vi "Colors.vi"() -> (0 "Highlight Color":u32(colorbox)=16776960, 1 "Text Color":u32(colorbox)=12303291, 2 "GridView Normal Color":u32(colorbox)=3618615, 3 "GridView Mouseover Color":u32(colorbox)=6645093)   [LabVIEW 2012, in "Win8uiFramework.lvlib"]
uses:
  Win8uiFramework/Win8uiFramework.lvlib
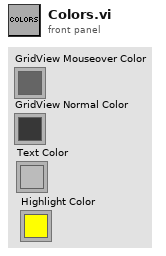
[diagram p1: front panel]
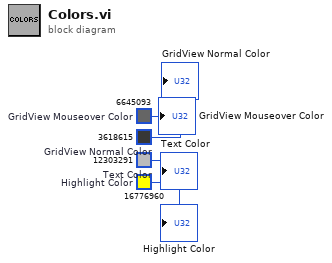
[diagram p0: block diagram]
diagram:
  w3 = u32 3618615  # GridView Normal Color
  w1 = u32 16776960  # Highlight Color
  w2 = u32 12303291  # Text Color
  w4 = u32 6645093  # GridView Mouseover Color
  "GridView Mouseover Color" <- w4
  "GridView Normal Color" <- w3
  "Text Color" <- w2
  "Highlight Color" <- w1
